vi "DataASCFileRichInfo.vi"(9 "Language":u32, 11 "file path (dialog if empty)":path caption="文件路径 （空时为对话框）") -> (0 "路径输出":path, 1 "FileInfo":string, 2 "文件类型":string)   [LabVIEW 2015]
uses:
  FileRichInfo2StringByTime.vi
  <vilib>/regexp/Match Regular Expression.xnode
panel:
  out "总帧数 2":i32
  out "倒数第二行":string
  out "判断":string
  out "倒数第一行":string
  out "第三行":string
  out "总帧数":i32
  out "第2行":string
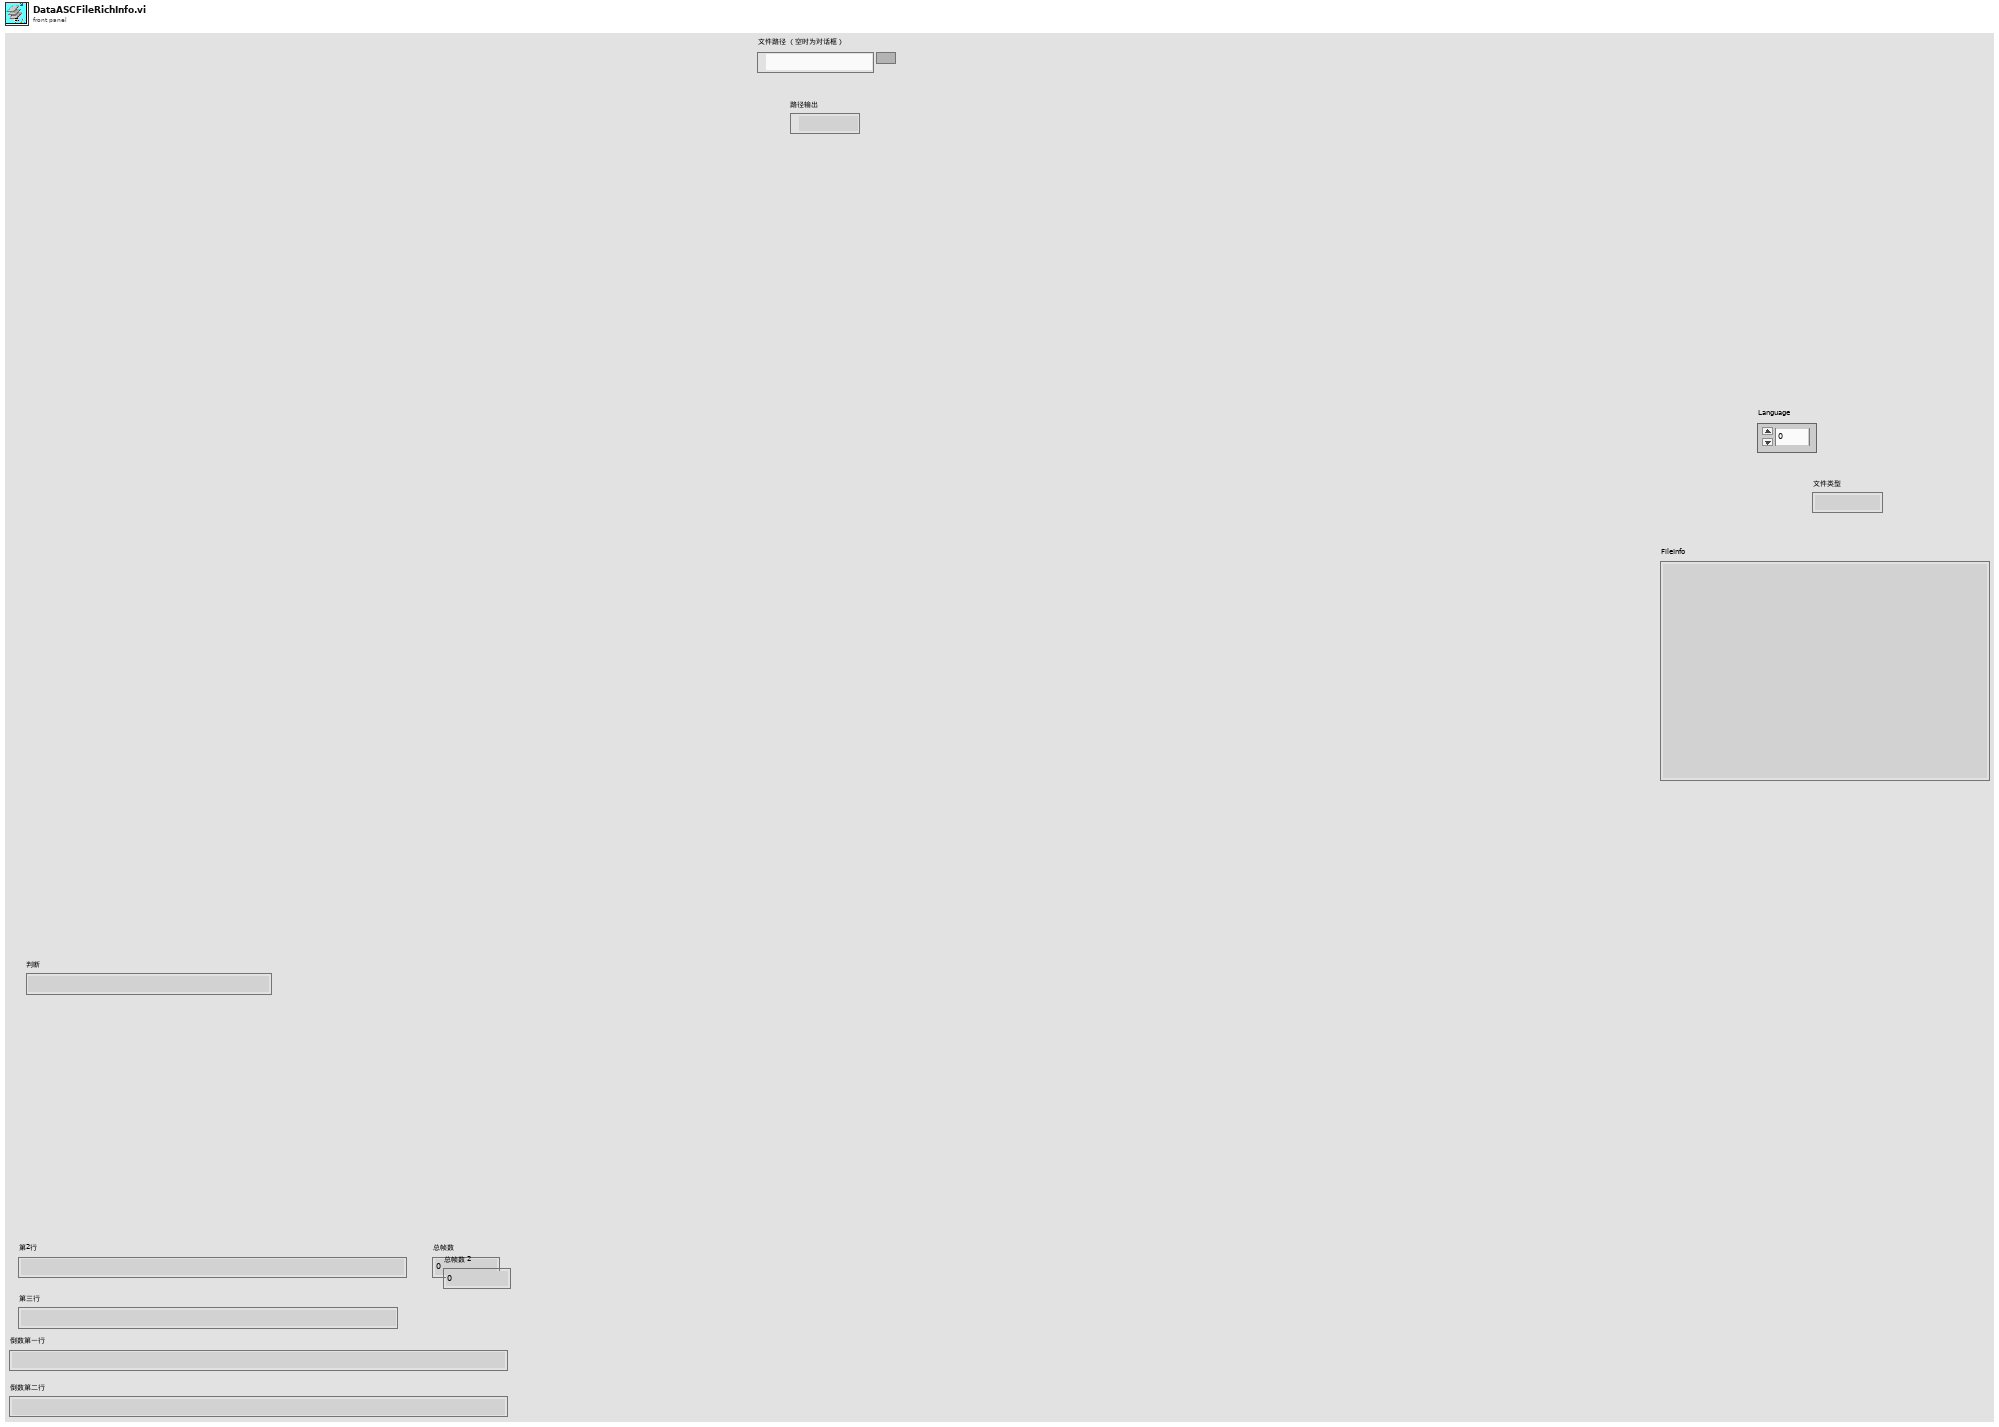
[diagram p1: front panel]
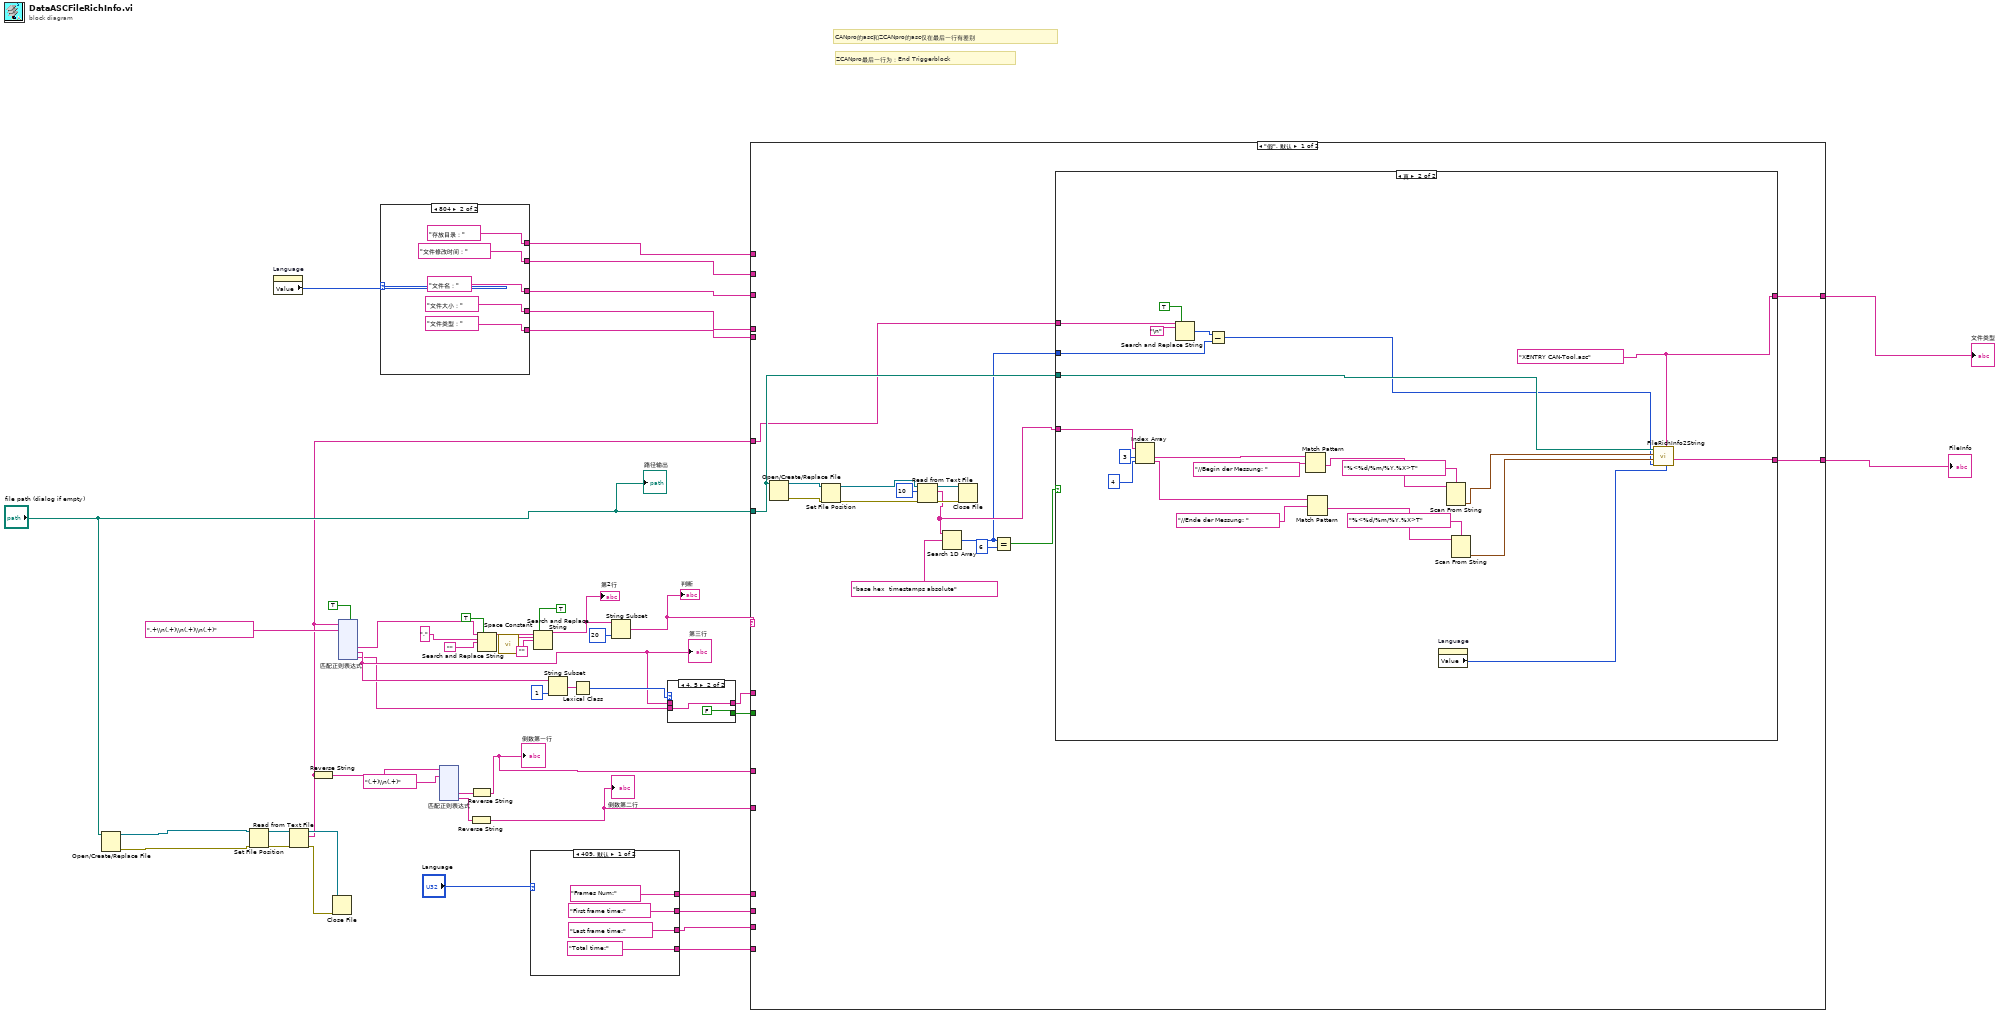
[diagram p0: block diagram]
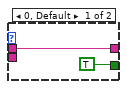
[diagram p2: hidden frame]
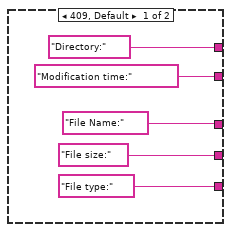
[diagram p3: hidden frame]
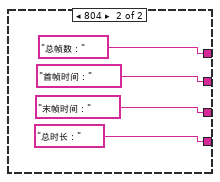
[diagram p4: hidden frame]
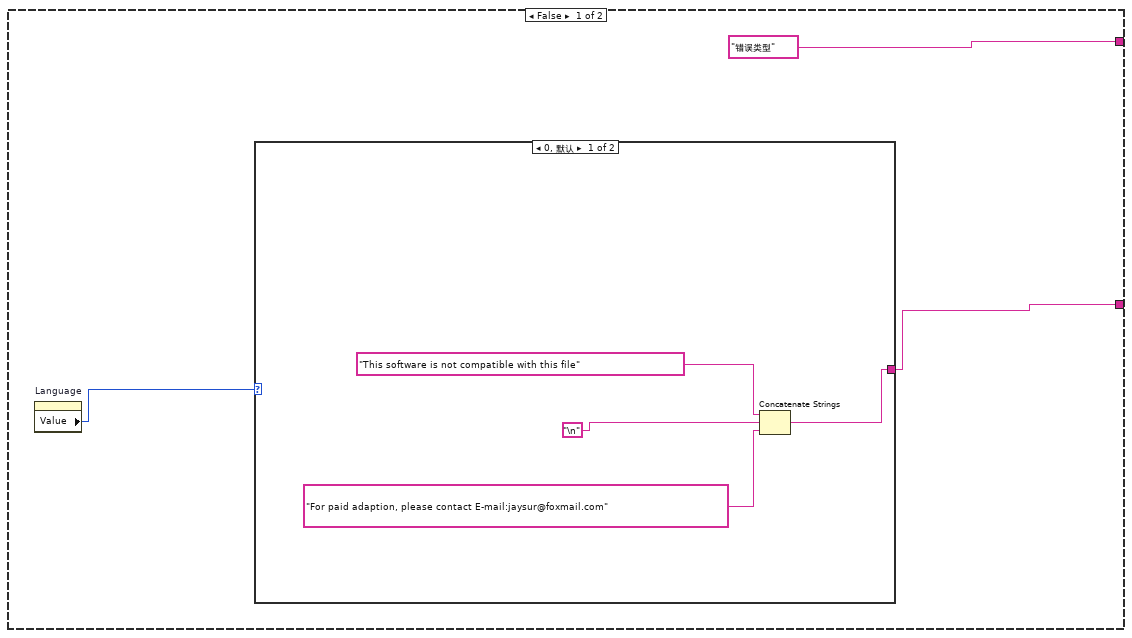
[diagram p5: hidden frame]
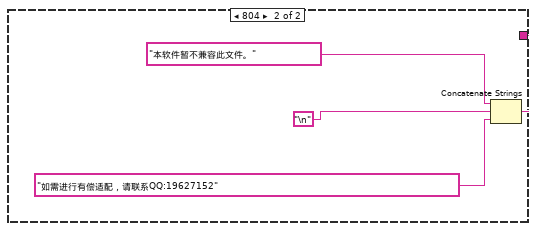
[diagram p6: hidden frame]
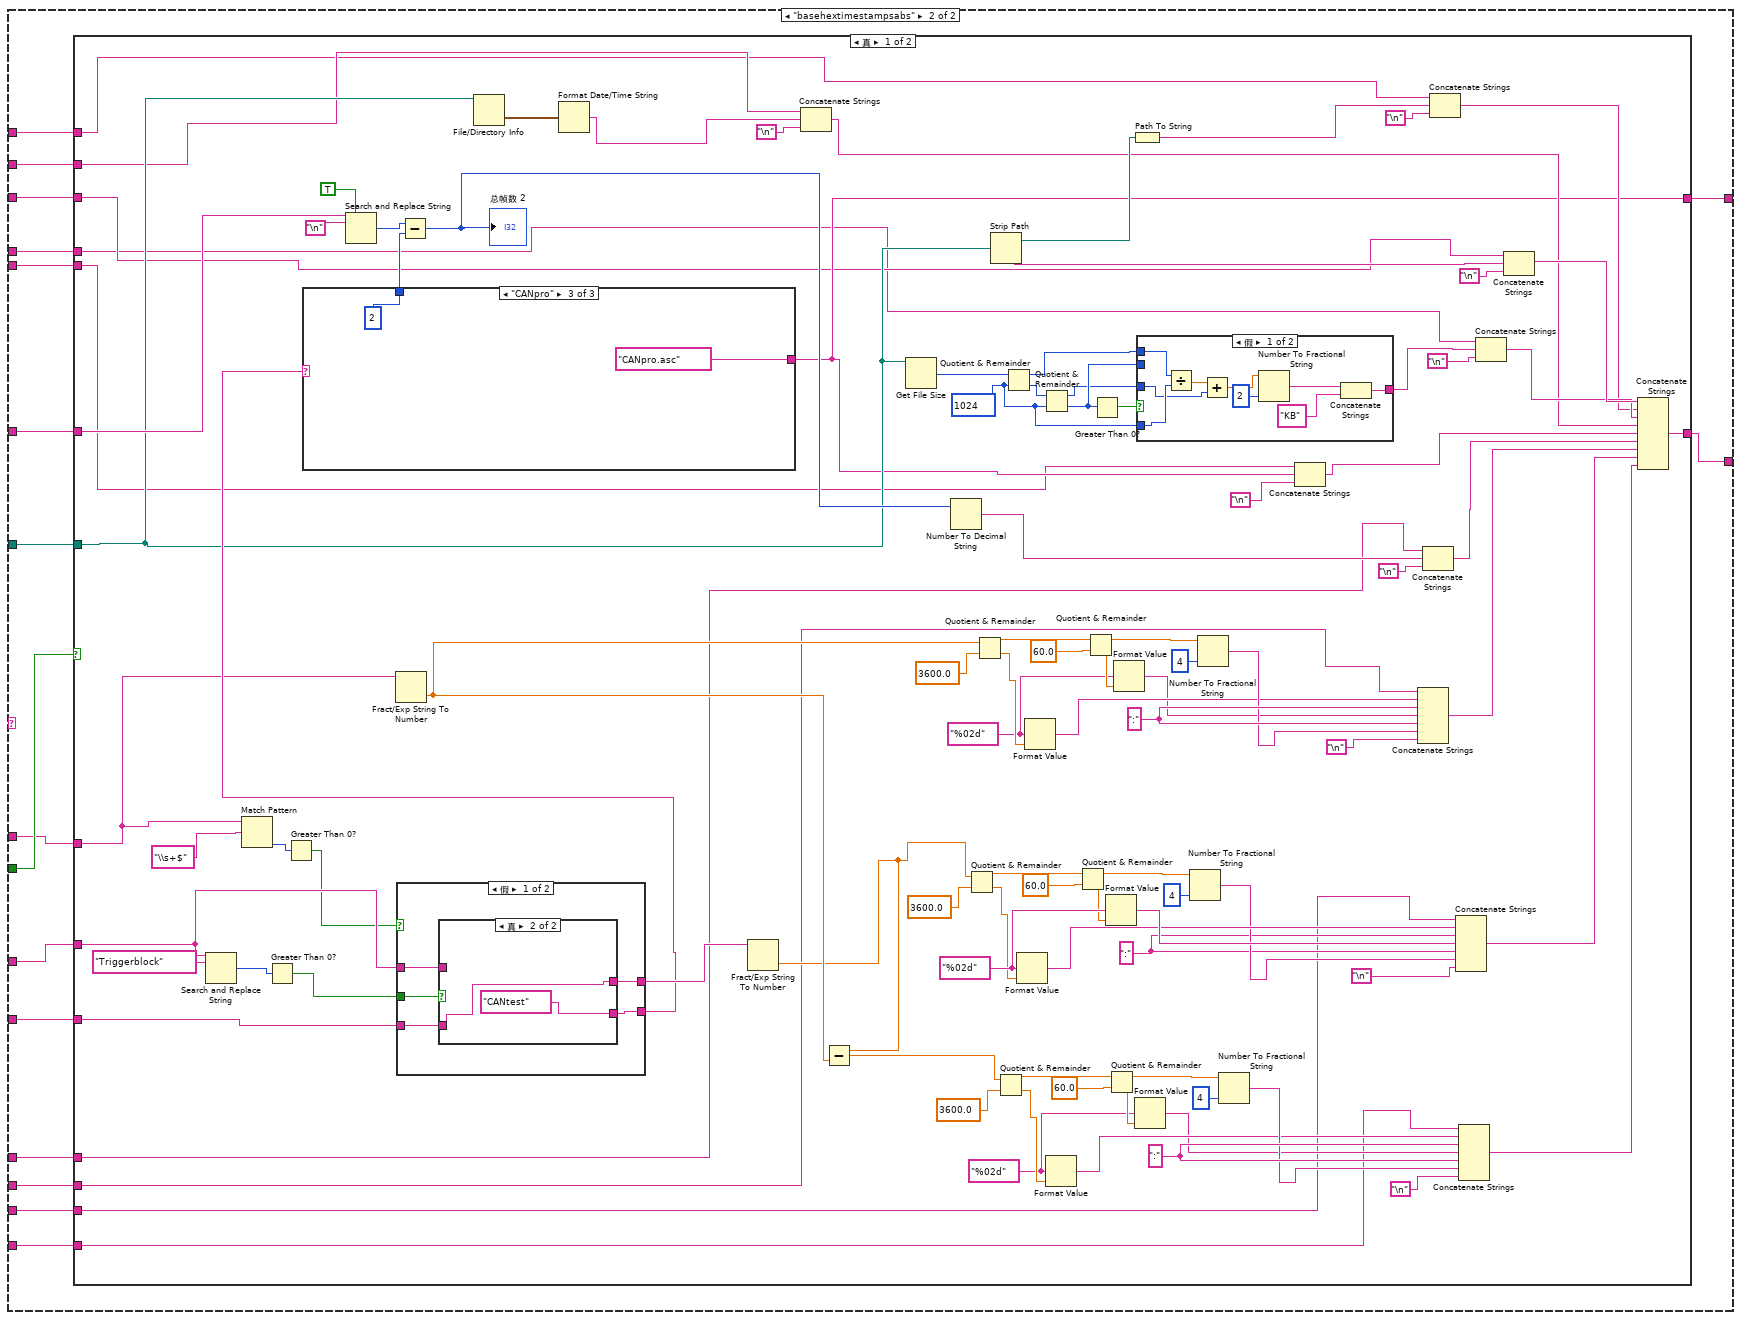
[diagram p7: hidden frame]
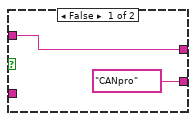
[diagram p8: hidden frame]
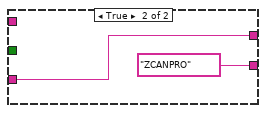
[diagram p9: hidden frame]
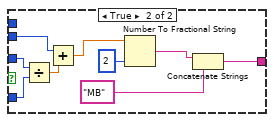
[diagram p10: hidden frame]
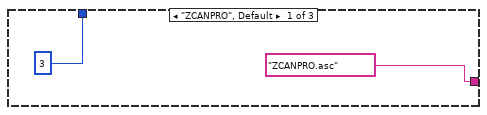
[diagram p11: hidden frame]
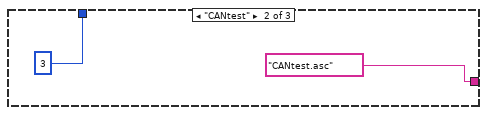
[diagram p12: hidden frame]
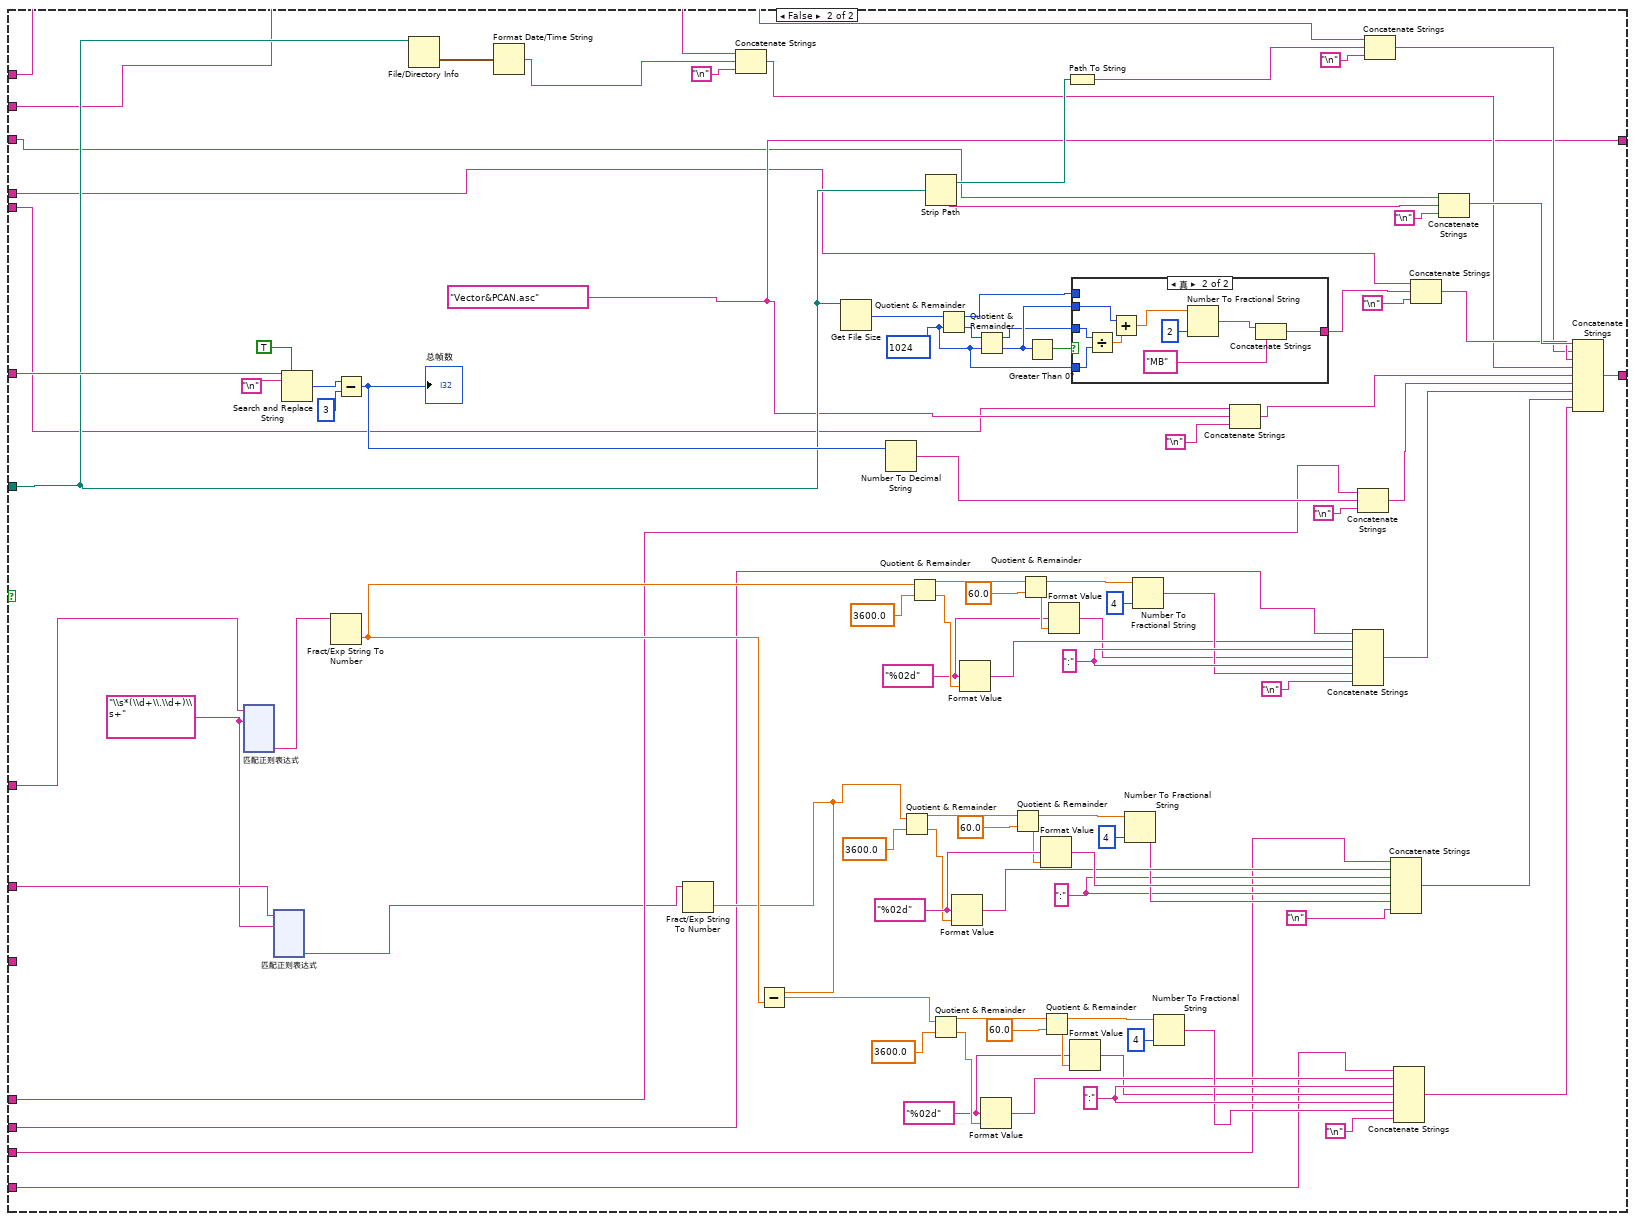
[diagram p13: hidden frame]
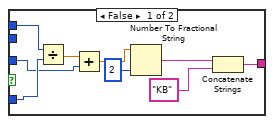
[diagram p14: hidden frame]
diagram:
  # "ZCANpro最后一行为：End Triggerblock"
  # "CANpro的asc和ZCANpro的asc仅在最后一行有差别"
  n1 = Open/Create/Replace File(file path (use dialog)="file path (dialog if empty)") -> (refnum out=w25:refnum<file>, error out=w24:errorcluster)  [unwired: 5 in, 1 out]
  n2 = Set File Position(refnum=w25, error in=w24) -> (refnum out=w45:refnum<file>, error out=w44:errorcluster)  [unwired: 2 in]
  n3 = property on="Language" class="DigNum (严格)"() -> ("Value"=w17:u32)  [unwired: 2 in, 2 out]
  n4 = Read from Text File(file (use dialog)=w45, error in=w44) -> (refnum out=w29:refnum<file>, text=w19:string, error out=w28:errorcluster)  [unwired: 2 in, 1 out]
  n5 = Reverse String(1:w19) -> (0:w33:string)
  n6 = Close File(refnum=w29, error in=w28) -> ()  [unwired: 2 out]
  n7 = xnode "匹配正则表达式"("输入字符串"=w19, "正则表达式"=".+\\n(.+)\\n(.+)\\n(.+)", "多行？(F)"=TRUE) -> ("子匹配 1"=w40:string, "子匹配 2"=w3:string, "子匹配 3"=w1:string)  [unwired: 3 in, 5 out]
  "第三行" <- w3
  n8 = case shown="804" w17 {
    tunnel: ["Modification time:" "文件修改时间："] -> w16
    tunnel: ["Directory:" "存放目录："] -> w13
    tunnel: ["File Name:" "文件名："] -> w14
    tunnel: ["File size:" "文件大小："] -> w12
    tunnel: ["File type:" "文件类型："] -> w15
    frame 409, Default {
    }
    frame 804 {
    }
  }
  n9 = xnode "匹配正则表达式"("输入字符串"=w33, "正则表达式"="(.+)\\n(.+)") -> ("子匹配 1"=w32:string, "子匹配 2"=w26:string)  [unwired: 4 in, 5 out]
  n10 = Reverse String(1:w26) -> (0:w21:string)
  "倒数第二行" <- w21
  n11 = Reverse String(1:w32) -> (0:w22:string)
  "倒数第一行" <- w22
  n12 = Search and Replace String(replace all?=TRUE ("替换全部？(F)"), input string=w40, search string=",", replace string="") -> (result string=w38:string)  [unwired: 4 in, 3 out]
  n13 = call <vilib>:"Space Constant.vi"() -> ("String"=w37:string)
  n14 = case shown="409, 默认" "Language" {
    tunnel: ["Total time:" "总时长："] -> w11
    tunnel: ["Last frame time:" "末帧时间："] -> w10
    tunnel: ["First frame time:" "首帧时间："] -> w9
    tunnel: ["Frames Num:" "总帧数："] -> w8
    frame 409, Default {
    }
    frame 804 {
    }
  }
  n15 = Search and Replace String(replace all?=TRUE ("替换全部？(F)"), input string=w38, search string=w37, replace string="") -> (result string=w31:string)  [unwired: 4 in, 3 out]
  "第2行" <- w31
  n16 = String Subset(string=w3, length (rest)=1 ("长度（剩余）")) -> (substring=w6:string)  [unwired: 1 in]
  n17 = Lexical Class(1:w6) -> (0:w5:i16)
  n18 = String Subset(string=w31, length (rest)=20 ("长度（剩余）")) -> (substring=w23:string)  [unwired: 1 in]
  "判断" <- w23
  n19 = case shown="4, 5" w5 {
    tunnel: [TRUE FALSE] -> w4
    tunnel: w3 -> [w66 _]
    tunnel: [w66 w68] -> w2
    tunnel: w1 -> [_ w68]
    frame 0, Default {
    }
    frame 4, 5 {
    }
  }
  n20 = case shown="\"假\", 默认" w23 {
    tunnel: [w85 w130] -> w47
    tunnel: [w84 w136] -> w46
    tunnel: "file path (dialog if empty)" -> [w72 w132]
    tunnel: w22 -> [_ w135]
    tunnel: w21 -> [_ w134]
    tunnel: w19 -> [w71 w133]
    tunnel: w16 -> [_ w131]
    tunnel: w15 -> [_ w129]
    tunnel: w14 -> [_ w128]
    tunnel: w13 -> [_ w127]
    tunnel: w12 -> [_ w126]
    tunnel: w11 -> [_ w125]
    tunnel: w10 -> [_ w124]
    tunnel: w9 -> [_ w123]
    tunnel: w8 -> [_ w122]
    tunnel: w4 -> [_ w121]
    tunnel: w2 -> [_ w120]
    frame "假", Default {
      n21 = Open/Create/Replace File(file path (use dialog)=w72) -> (refnum out=w80:refnum<file>, error out=w79:errorcluster)  [unwired: 5 in, 1 out]
      n22 = Set File Position(refnum=w80, error in=w79) -> (refnum out=w77:refnum<file>, error out=w78:errorcluster)  [unwired: 2 in]
      n23 = Read from Text File(file (use dialog)=w77, count=10 ("计数"), error in=w78) -> (refnum out=w82:refnum<file>, text=w73:string[], error out=w83:errorcluster)  [unwired: 1 in, 1 out]
      n24 = Search 1D Array(1D array=w73, element="base hex  timestamps absolute") -> (index of element=w70:i32)  [unwired: 1 in]
      n25 = Close File(refnum=w82, error in=w83) -> ()  [unwired: 2 out]
      n26 = Equal?(x=w70, y=6) -> (x = y?=w74:bool)
      n27 = case shown="真" w74 {
        tunnel: ["错误类型" w97] -> w85
        tunnel: [w87 w98] -> w84
        tunnel: w73 -> [_ w113]
        tunnel: w72 -> [_ w102]
        tunnel: w71 -> [_ w109]
        tunnel: w70 -> [_ w108]
        frame False {
          n28 = property on="Language" class="DigNum (严格)"() -> ("Value"=w86:u32)  [unwired: 2 in, 2 out]
          n29 = case shown="0, 默认" w86 {
            tunnel: [w89 w93] -> w87
            frame 0, Default {
              n30 = Concatenate Strings("This software is not compatible with this file", "\n", "For paid adaption, please contact E-mail:jaysur@foxmail.com") -> (w89:string)
            }
            frame 804 {
              n31 = Concatenate Strings("本软件暂不兼容此文件。", "\n", "如需进行有偿适配，请联系QQ:19627152") -> (w93:string)
            }
          }
        }
        frame True {
          w97 = "XENTRY CAN-Tool.asc" ("文件类型")
          n32 = Index Array(array=w113, index #1=3 ("索引"), index #2=4 ("索引")) -> (element #1=w117:string, element #2=w115:string)
          n33 = Search and Replace String(replace all?=TRUE ("替换全部？(F)"), input string=w109, search string="\n") -> (number of replacements=w111:i32)  [unwired: 5 in, 3 out]
          n34 = Subtract(x=w111, y=w108) -> (x-y=w99:i32)
          n35 = Match Pattern(string=w117, regular expression="//Begin der Messung: " ("正则表达式")) -> (after substring=w104:string)  [unwired: 1 in, 3 out]
          n36 = Match Pattern(string=w115, regular expression="//Ende der Messung: " ("正则表达式")) -> (after substring=w106:string)  [unwired: 1 in, 3 out]
          n37 = property on="Language" class="DigNum (严格)"() -> ("Value"=w103:u32)  [unwired: 2 in, 2 out]
          n38 = Scan From String(format string="%<%d/%m/%Y,%X>T" ("格式字符串"), input string=w104) -> (output 1=w101:timestamp)  [unwired: 3 in, 3 out]
          n39 = Scan From String(format string="%<%d/%m/%Y,%X>T" ("格式字符串"), input string=w106) -> (output 1=w100:timestamp)  [unwired: 3 in, 3 out]
          n40 = call-poly "FileRichInfo2String.vi"("file path (dialog if empty)"=w102, "BeginTime"=w101, "EndTime"=w100, "总帧数"=w99, "文件类型"=w97, "Language"=w103) -> ("FileInfo"=w98:string)  [unwired: 3 in]
        }
      }
    }
    frame "basehextimestampsabs" {
      n41 = case shown="真" w121 {
        tunnel: [w224 w353] -> w136
        tunnel: w135 -> [w171 w274]
        tunnel: w134 -> [w168 _]
        tunnel: w133 -> [w163 w298]
        tunnel: w120 -> [w159 w276]
        tunnel: w132 -> [w148 w288]
        tunnel: w131 -> [w146 w286]
        tunnel: [w145 w285] -> w130
        tunnel: w129 -> [w144 w284]
        tunnel: w128 -> [w143 w283]
        tunnel: w127 -> [w142 w282]
        tunnel: w126 -> [w141 w281]
        tunnel: w125 -> [w140 w280]
        tunnel: w124 -> [w139 w279]
        tunnel: w123 -> [w138 w278]
        tunnel: w122 -> [w137 w277]
        frame True {
          w179 = i64 1024 ("y")
          w198 = "%02d" ("格式字符串")
          w204 = ":"
          w222 = "%02d" ("格式字符串")
          w216 = ":"
          w225 = "%02d" ("格式字符串")
          w231 = ":"
          n42 = Search and Replace String(input string=w171, search string="Triggerblock" ("搜索字符串")) -> (number of replacements=w173:i32)  [unwired: 6 in, 3 out]
          n43 = Match Pattern(string=w159, regular expression="\\s+$") -> (offset past match=w158:i32)  [unwired: 1 in, 3 out]
          n44 = Greater Than 0?(x=w173) -> (x > 0?=w156:bool)
          n45 = Greater Than 0?(x=w158) -> (x > 0?=w157:bool)
          n46 = Search and Replace String(replace all?=TRUE ("替换全部？(F)"), input string=w163, search string="\n") -> (number of replacements=w165:i32)  [unwired: 5 in, 3 out]
          n47 = Fract/Exp String To Number(string=w159) -> (number=w174:dbl)  [unwired: 3 in, 1 out]
          n48 = case shown="假" w157 {
            tunnel: [w240 w247] -> w170
            tunnel: w168 -> [w237 w247]
            tunnel: [w241 "ZCANPRO"] -> w167
            tunnel: w171 -> [w239 _]
            tunnel: w156 -> [w238 _]
            frame False {
              n49 = case shown="真" w238 {
                tunnel: ["CANpro" "CANtest"] -> w241
                tunnel: [w242 w245] -> w240
                tunnel: w239 -> [w242 _]
                tunnel: w237 -> [_ w245]
                frame False {
                }
                frame True {
                }
              }
            }
            frame True {
            }
          }
          n50 = case shown="\"CANpro\"" w167 {
            tunnel: ["ZCANPRO.asc" "CANtest.asc" "CANpro.asc"] -> w145
            tunnel: [3 ("y") 3 ("y") 2 ("y")] -> w162
            frame "ZCANPRO", Default {
            }
            frame "CANtest" {
            }
            frame "CANpro" {
            }
          }
          n51 = Subtract(x=w165, y=w162) -> (x-y=w161:i32)
          "总帧数 2" <- w161
          n52 = File/Directory Info(path=w148) -> (last mod=w151:timestamp)  [unwired: 1 in, 6 out]
          n53 = Format Date/Time String(seconds (now)=w151) -> (date/time string=w149:string)  [unwired: 2 in]
          n54 = Fract/Exp String To Number(string=w170) -> (number=w169:dbl)  [unwired: 3 in, 1 out]
          n55 = Concatenate Strings(w146, w149, "\n") -> (w147:string)
          n56 = Subtract(x=w169, y=w174) -> (x-y=w197:dbl)
          n57 = Get File Size(file=w148) -> (size (in bytes)=w182:i64)  [unwired: 1 in, 2 out]
          n58 = Number To Decimal String(number=w161) -> (decimal integer string=w185:string)  [unwired: 1 in]
          n59 = Quotient & Remainder(x=w169, y=3600.0) -> (x-y*floor(x/y)=w212:dbl, floor(x/y)=w219:dbl)
          n60 = Quotient & Remainder(x=w174, y=3600.0) -> (x-y*floor(x/y)=w235:dbl, floor(x/y)=w228:dbl)
          n61 = Strip Path(path=w148) -> (stripped path=w153:path, name=w192:string)
          n62 = Quotient & Remainder(x=w197, y=3600.0) -> (x-y*floor(x/y)=w208:dbl, floor(x/y)=w201:dbl)
          n63 = Quotient & Remainder(x=w182, y=w179) -> (x-y*floor(x/y)=w175:i64, floor(x/y)=w181:i64)
          n64 = Format Value(format string=w222, value (0)=w219) -> (output string=w218:string)  [unwired: 1 in]
          n65 = Format Value(format string=w225, value (0)=w228) -> (output string=w229:string)  [unwired: 1 in]
          n66 = Quotient & Remainder(x=w181, y=w179) -> (x-y*floor(x/y)=w177:i64, floor(x/y)=w178:i64)
          n67 = Format Value(format string=w198, value (0)=w201) -> (output string=w202:string)  [unwired: 1 in]
          n68 = Quotient & Remainder(x=w212, y=60.0) -> (x-y*floor(x/y)=w214:dbl, floor(x/y)=w220:dbl)
          n69 = Quotient & Remainder(x=w235, y=60.0) -> (x-y*floor(x/y)=w233:dbl, floor(x/y)=w227:dbl)
          n70 = Greater Than 0?(x=w178) -> (x > 0?=w180:bool)
          n71 = Format Value(format string=w222, value (0)=w220) -> (output string=w221:string)  [unwired: 1 in]
          n72 = Quotient & Remainder(x=w208, y=60.0) -> (x-y*floor(x/y)=w206:dbl, floor(x/y)=w200:dbl)
          n73 = Format Value(format string=w225, value (0)=w227) -> (output string=w226:string)  [unwired: 1 in]
          n74 = Path To String(path=w153) -> (string=w154:string)
          n75 = Format Value(format string=w198, value (0)=w200) -> (output string=w199:string)  [unwired: 1 in]
          n76 = case shown="假" w180 {
            tunnel: w179 -> [w253 w263]
            tunnel: w178 -> [_ w261]
            tunnel: w177 -> [w251 w264]
            tunnel: [w256 w259] -> w176
            tunnel: w175 -> [w254 _]
            frame False {
              n77 = Divide(x=w254, y=w253) -> (x/y=w252:dbl)
              n78 = Add(x=w252, y=w251) -> (x+y=w250:dbl)
              n79 = Number To Fractional String(number=w250, precision (6)=i16 2 ("精度(6)")) -> (F-format string=w248:string)  [unwired: 2 in]
              n80 = Concatenate Strings(w248, "KB" ("字符串")) -> (w256:string)
            }
            frame True {
              n81 = Divide(x=w264, y=w263) -> (x/y=w262:dbl)
              n82 = Add(x=w261, y=w262) -> (x+y=w260:dbl)
              n83 = Number To Fractional String(number=w260, precision (6)=i16 2 ("精度(6)")) -> (F-format string=w258:string)  [unwired: 2 in]
              n84 = Concatenate Strings(w258, "MB") -> (w259:string)
            }
          }
          n85 = Number To Fractional String(number=w214, precision (6)=i16 4 ("精度(6)")) -> (F-format string=w217:string)  [unwired: 2 in]
          n86 = Number To Fractional String(number=w233, precision (6)=i16 4 ("精度(6)")) -> (F-format string=w230:string)  [unwired: 2 in]
          n87 = Number To Fractional String(number=w206, precision (6)=i16 4 ("精度(6)")) -> (F-format string=w203:string)  [unwired: 2 in]
          n88 = Concatenate Strings(w144, w145, "\n") -> (w189:string)
          n89 = Concatenate Strings(w138, w229, w231, w226, w231, w230, "\n") -> (w223:string)
          n90 = Concatenate Strings(w137, w185, "\n") -> (w186:string)
          n91 = Concatenate Strings(w142, w154, "\n") -> (w152:string)
          n92 = Concatenate Strings(w139, w218, w216, w221, w216, w217, "\n") -> (w210:string)
          n93 = Concatenate Strings(w140, w202, w204, w199, w204, w203, "\n") -> (w196:string)
          n94 = Concatenate Strings(w141, w176, "\n") -> (w183:string)
          n95 = Concatenate Strings(w143, w192, "\n") -> (w191:string)
          n96 = Concatenate Strings(w191, w152, w183, w147, w189, w186, w223, w210, w196) -> (w224:string)
        }
        frame False {
          w273 = "\\s*(\\d+\\.\\d+)\\s+" ("正则表达式")
          w285 = "Vector&PCAN.asc"
          w308 = i64 1024 ("y")
          w327 = "%02d" ("格式字符串")
          w333 = ":"
          w351 = "%02d" ("格式字符串")
          w345 = ":"
          w354 = "%02d" ("格式字符串")
          w360 = ":"
          n97 = xnode "匹配正则表达式"("输入字符串"=w276, "正则表达式"=w273) -> ("子匹配 1"=w275:string)  [unwired: 4 in, 5 out]
          n98 = xnode "匹配正则表达式"("输入字符串"=w274, "正则表达式"=w273) -> ("子匹配 1"=w272:string)  [unwired: 4 in, 5 out]
          n99 = Search and Replace String(replace all?=TRUE ("替换全部？(F)"), input string=w298, search string="\n") -> (number of replacements=w300:i32)  [unwired: 5 in, 3 out]
          n100 = Fract/Exp String To Number(string=w275) -> (number=w303:dbl)  [unwired: 3 in, 1 out]
          n101 = Subtract(x=w300, y=3) -> (x-y=w296:i32)
          "总帧数" <- w296
          n102 = File/Directory Info(path=w288) -> (last mod=w291:timestamp)  [unwired: 1 in, 6 out]
          n103 = Format Date/Time String(seconds (now)=w291) -> (date/time string=w289:string)  [unwired: 2 in]
          n104 = Fract/Exp String To Number(string=w272) -> (number=w302:dbl)  [unwired: 3 in, 1 out]
          n105 = Concatenate Strings(w286, w289, "\n") -> (w287:string)
          n106 = Subtract(x=w302, y=w303) -> (x-y=w326:dbl)
          n107 = Get File Size(file=w288) -> (size (in bytes)=w311:i64)  [unwired: 1 in, 2 out]
          n108 = Number To Decimal String(number=w296) -> (decimal integer string=w314:string)  [unwired: 1 in]
          n109 = Quotient & Remainder(x=w302, y=3600.0) -> (x-y*floor(x/y)=w341:dbl, floor(x/y)=w348:dbl)
          n110 = Quotient & Remainder(x=w303, y=3600.0) -> (x-y*floor(x/y)=w364:dbl, floor(x/y)=w357:dbl)
          n111 = Strip Path(path=w288) -> (stripped path=w293:path, name=w321:string)
          n112 = Quotient & Remainder(x=w326, y=3600.0) -> (x-y*floor(x/y)=w337:dbl, floor(x/y)=w330:dbl)
          n113 = Quotient & Remainder(x=w311, y=w308) -> (x-y*floor(x/y)=w304:i64, floor(x/y)=w310:i64)
          n114 = Format Value(format string=w351, value (0)=w348) -> (output string=w347:string)  [unwired: 1 in]
          n115 = Format Value(format string=w354, value (0)=w357) -> (output string=w358:string)  [unwired: 1 in]
          n116 = Quotient & Remainder(x=w310, y=w308) -> (x-y*floor(x/y)=w306:i64, floor(x/y)=w307:i64)
          n117 = Format Value(format string=w327, value (0)=w330) -> (output string=w331:string)  [unwired: 1 in]
          n118 = Quotient & Remainder(x=w341, y=60.0) -> (x-y*floor(x/y)=w343:dbl, floor(x/y)=w349:dbl)
          n119 = Quotient & Remainder(x=w364, y=60.0) -> (x-y*floor(x/y)=w362:dbl, floor(x/y)=w356:dbl)
          n120 = Greater Than 0?(x=w307) -> (x > 0?=w309:bool)
          n121 = Format Value(format string=w351, value (0)=w349) -> (output string=w350:string)  [unwired: 1 in]
          n122 = Quotient & Remainder(x=w337, y=60.0) -> (x-y*floor(x/y)=w335:dbl, floor(x/y)=w329:dbl)
          n123 = Format Value(format string=w354, value (0)=w356) -> (output string=w355:string)  [unwired: 1 in]
          n124 = Path To String(path=w293) -> (string=w294:string)
          n125 = Format Value(format string=w327, value (0)=w329) -> (output string=w328:string)  [unwired: 1 in]
          n126 = case shown="真" w309 {
            tunnel: w308 -> [w603 w613]
            tunnel: w307 -> [_ w611]
            tunnel: w306 -> [w601 w614]
            tunnel: [w606 w609] -> w305
            tunnel: w304 -> [w604 _]
            frame False {
              n127 = Divide(x=w604, y=w603) -> (x/y=w602:dbl)
              n128 = Add(x=w602, y=w601) -> (x+y=w600:dbl)
              n129 = Number To Fractional String(number=w600, precision (6)=i16 2 ("精度(6)")) -> (F-format string=w598:string)  [unwired: 2 in]
              n130 = Concatenate Strings(w598, "KB" ("字符串")) -> (w606:string)
            }
            frame True {
              n131 = Divide(x=w614, y=w613) -> (x/y=w612:dbl)
              n132 = Add(x=w611, y=w612) -> (x+y=w610:dbl)
              n133 = Number To Fractional String(number=w610, precision (6)=i16 2 ("精度(6)")) -> (F-format string=w608:string)  [unwired: 2 in]
              n134 = Concatenate Strings(w608, "MB") -> (w609:string)
            }
          }
          n135 = Number To Fractional String(number=w343, precision (6)=i16 4 ("精度(6)")) -> (F-format string=w346:string)  [unwired: 2 in]
          n136 = Number To Fractional String(number=w362, precision (6)=i16 4 ("精度(6)")) -> (F-format string=w359:string)  [unwired: 2 in]
          n137 = Number To Fractional String(number=w335, precision (6)=i16 4 ("精度(6)")) -> (F-format string=w332:string)  [unwired: 2 in]
          n138 = Concatenate Strings(w284, w285, "\n") -> (w318:string)
          n139 = Concatenate Strings(w278, w358, w360, w355, w360, w359, "\n") -> (w352:string)
          n140 = Concatenate Strings(w277, w314, "\n") -> (w315:string)
          n141 = Concatenate Strings(w282, w294, "\n") -> (w292:string)
          n142 = Concatenate Strings(w279, w347, w345, w350, w345, w346, "\n") -> (w339:string)
          n143 = Concatenate Strings(w280, w331, w333, w328, w333, w332, "\n") -> (w325:string)
          n144 = Concatenate Strings(w281, w305, "\n") -> (w312:string)
          n145 = Concatenate Strings(w283, w321, "\n") -> (w320:string)
          n146 = Concatenate Strings(w320, w292, w312, w287, w318, w315, w352, w339, w325) -> (w353:string)
        }
      }
    }
  }
  "FileInfo" <- w46
  "文件类型" <- w47
  "路径输出" <- "file path (dialog if empty)"
